vi "Window Handle Manager.vi"(8 "Force Close?":bool, 10 "Container State":T1, 11 "Display State in":T2={"Window Handle"=refnum, "Maximum"=0, "State Change Action"=enum."Method - Initialize", "Running"=FALSE, "Visable Items"={"Label"=TRUE, "Caption"=FALSE}, "Value"=100, "Show Progress Bar"=FALSE} caption="State") -> (3 "Display State out":T2={"Window Handle"=refnum, "Maximum"=0, "State Change Action"=enum."Method - Initialize", "Running"=FALSE, "Visable Items"={"Label"=TRUE, "Caption"=FALSE}, "Value"=100, "Show Progress Bar"=FALSE} caption="State")   [LabVIEW 2011, in "Taskbar Progress Bar.xctl"]
uses:
  Taskbar Progress Bar.xctl
  Abilities/TPB State.ctl
  TypeDefs/Dispaly State Change Methods.ctl
  <vilib>/_xctls/Container State.ctl
  <vilib>/TaskbarProgressAPI/_TypeDefs/Progress State.ctl
  <vilib>/TaskbarProgressAPI/TaskbarProgressAPI.lvlib
  <vilib>/_xctls/XControlSupport.lvlib
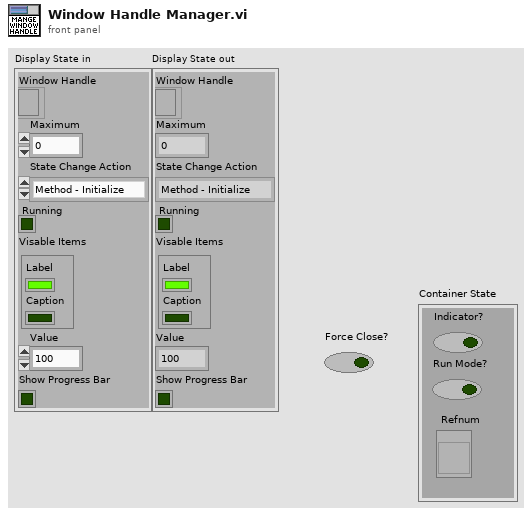
[diagram p1: front panel]
types:
  T1 = typedef "XControlSupport.lvlib/Container State.ctl" = cluster{"Indicator?":bool, "Run Mode?":bool, " Refnum":refnum<vi>}
  T2 = typedef "Taskbar Progress Bar.xctl/TPB State.ctl" = cluster{"Window Handle":refnum<k24>, "Maximum":u64, "State Change Action":T3, "Running":bool, "Visable Items":cluster{"Label":bool, "Caption":bool}, "Value":u64, "Show Progress Bar":bool}
  T3 = typedef "Taskbar Progress Bar.xctl/Dispaly State Change Methods.ctl" = enum16{"No Action", "Created", "Method - Initialize", "Method - Increment", "Method - Set Value", "Method - Pause", "Method - Error", "Method - Finish", "Property - Show Progress Bar"}
  T4 = typedef "TaskbarProgressAPI.lvlib/Progress State.ctl" = i32
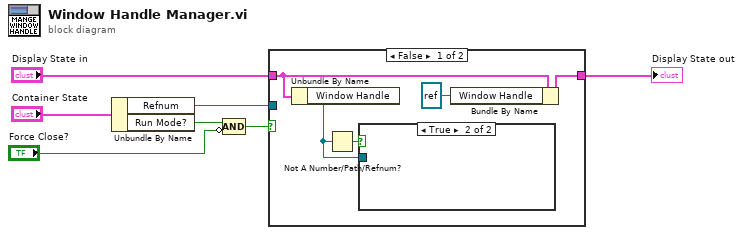
[diagram p0: block diagram]
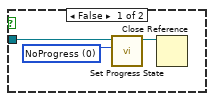
[diagram p2: hidden frame]
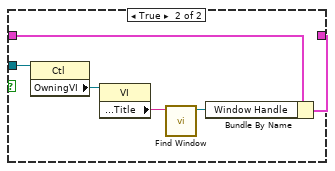
[diagram p3: hidden frame]
diagram:
  n1 = Unbundle By Name("Container State") -> ("Refnum"=w6:refnum<vi>, "Run Mode?"=w3:bool)
  n2 = Compound Arithmetic op=AND(w3, invert "Force Close?") -> (w2:bool)
  n3 = case shown="False" w2 {
    tunnel: "Display State in" -> [w10 w18]
    tunnel: w6 -> [_ w21]
    tunnel: [w9 w17] -> w7
    frame False {
      n4 = Unbundle By Name(w10) -> ("Window Handle"=w11:refnum<k24>)
      n5 = Not A Number/Path/Refnum?(number/path/refnum=w11) -> (NaN/Path/Refnum?=w12:bool)
      n6 = case shown="True" w12 {
        tunnel: w11 -> [w15 _]
        frame False {
          w14 = T4 0 items=["NoProgress"=0, "Indeterminate"=1, "Normal"=2, "Error"=4, "Paused"=8] ("State (No Progress)")
          n7 = call <vilib>:"Set Progress State.vi"("State (No Progress)"=w14, "Window Handle"=w15) -> ("dup Window Handle"=w13:refnum<k24>)  [unwired: 8 in, 1 out]
          n8 = Close Reference(reference=w13) -> ()  [unwired: 1 in, 1 out]
        }
        frame True {
        }
      }
      n9 = Bundle By Name(cluster=w10, "Window Handle"=refnum<k24> refnum) -> (w9:T2)
    }
    frame True {
      n10 = property class="Ctl"(reference=w21) -> ("OwningVI"=w20:refnum<vi>)  [unwired: 1 in, 2 out]
      n11 = property class="VI"(reference=w20) -> ("Front Panel.Title"=w19:string)  [unwired: 1 in, 2 out]
      n12 = call <vilib>:"Find Window.vi"("Window Title (Callers Window)"=w19) -> ("Window Handle"=w16:refnum<k24>)  [unwired: 9 in, 1 out]
      n13 = Bundle By Name(cluster=w18, "Window Handle"=w16) -> (w17:T2)
    }
  }
  "Display State out" <- w7
